vi "ESR Scanner - modified.vi"(0 "ESR Modified Parameters":T5={"Window 1 time (s)"=0.012, "Window 2 time (s)"=5e-06, "Window 3 time (s) "=0.02, "Window 4 time (s)"=5e-07, "Window 4 channels"=[TRUE, FALSE, FALSE, TRUE], "Window 3 channels"=[TRUE, FALSE, TRUE, TRUE], "Window 2 channels"=[TRUE, FALSE, FALSE, TRUE], "Window 1 channels"=[TRUE, TRUE, FALSE, TRUE], "Path to ESR Burner"=path "C:/Users/Loncar/Desktop/ESR VIs - Srujan/Sam Kim/PB/ESRFreq.exe", "Window 5 time (s)"=5e-07, "Drive channel"=0} {"Drive channel" max=8}, 1 "MW start freq (GHz)":dbl=2.84, 2 "MW stop freq (GHz)":dbl=2.9, 3 "# freq points":i32=61, 4 "# scans before track":i32=50, 5 "#scan iterations":i32=50, 6 "IntGraph Refnum":refnum<vi>, 7 "Optimize Parameters":T6={"Volt Step"={"X"=0.01, "Y"=0.01, "Z"=0.0}, "Num Iterations"=1, "Dwell Time (ms)"=100, "Volts Range"={"X"=0.1, "Y"=0.1, "Z"=0.0}, "Method"={"X"=enum."Max", "Y"=enum."Max", "Z"=enum."Max"}} {"Volts Range"."Z" min=0.0; "Volts Range"."Y" min=0.0; "Volts Range"."X" min=0.0; "Dwell Time (ms)" min=0; "Num Iterations" min=1 step=1; "Volt Step"."Z" min=1e-05; "Volt Step"."Y" min=1e-06; "Volt Step"."X" min=1e-06}, 8 "XY Graph Refnum":refnum<vi>, 9 "ESR Post-Processing Parameters":T3={"Cut-off Threshhold"=2.0, "Processing Type"=enum."Off"}, 10 "IntGraph Refnum 2":refnum<vi>, 11 "Data 1":T1={"Save avg spectrum graph?"=FALSE, "Path for avg spectrum graph"=path "C:/experiment/data/may_15_2012/SIL1_NV1_pippin_uW_off", "Save data to spreadsheet"=FALSE, "Path for avg spectrum spreadsheet"=path "C:/experiment/data/may_15_2012/SIL1_NV1_pippin_uW_off"}, 12 "XY Graph Refnum 2":refnum<vi>, 13 "Data 2":T2={"Save graph 2"=FALSE, "Path for avg spectrum graph 2"=path "C:/experiment/data/may_15_2012/SIL1_NV1_pippin_uW_off", "Save data to spreadsheet 2"=FALSE, "Path for avg spectrum spreadsheet 2"=path "C:/experiment/data/may_15_2012/SIL1_NV1_pippin_uW_off"}) -> ()   [LabVIEW 2012]
uses:
  Strict Type Def - Optimize Parameters Cluster.ctl
  ESR Modified Window Parameters.ctl
  ESR Processing Params.ctl
  ESR Processing State.ctl
  <vilib>/DAQmx/read.llb/DAQmx Read (Counter 1D U32 1Chan NSamp).vi
  Channels.vi
  <vilib>/DAQmx/miscellaneous.llb/DAQmx Fill In Error Info.vi
  Global Vars.vi
  <vilib>/Analysis/baseanly.llb/Mean (DBL).vi
  <vilib>/Utility/file.llb/Write To Spreadsheet File (DBL).vi
  <vilib>/Analysis/NI_AALBase.lvlib
panel:
  out "Counts vs. frequency 2":i32[][](graph)
  out "Avg ESR spectrum 2":cluster{"Y":dbl[], "Y":dbl[]}[](graph)
  out "Counts vs. frequency before processing":i32[][](graph)
  out "Counts vs. frequency":i32[][](graph)
  out "Avg ESR spectrum":cluster{"Y":dbl[], "Y":dbl[]}[](graph)
  # "Note:\nThis is not a standalone program. It is called from ScannerUI"
  # "Default PB connections:\nPB0 - MW switch\nPB1 - MW freq step\nPB2 - Counter sample clk\nPB3 - Green AOM"
  # "VI for ESR spectrum measurement\n08/26/2013, Srujan Meesala\n2/2/2015, Samuel Kim"
  # "Modified version:\nAlternates frequency sweep with channel on/off for driving cantilever"
  # "this is for each, ie 50 scans =\n50 scans off + 50 scans on"
  # "* <data>"
  # "MW freq step\ndwell time"
  # "MW freq step"
  # "Wait"
  # "Fluorescence\ncounting"
  # "Ctr sample clk"
  # "Wait"
  # "Wait between\nfreq sweeps"
  # "On/off between freq sweeps (off first)"
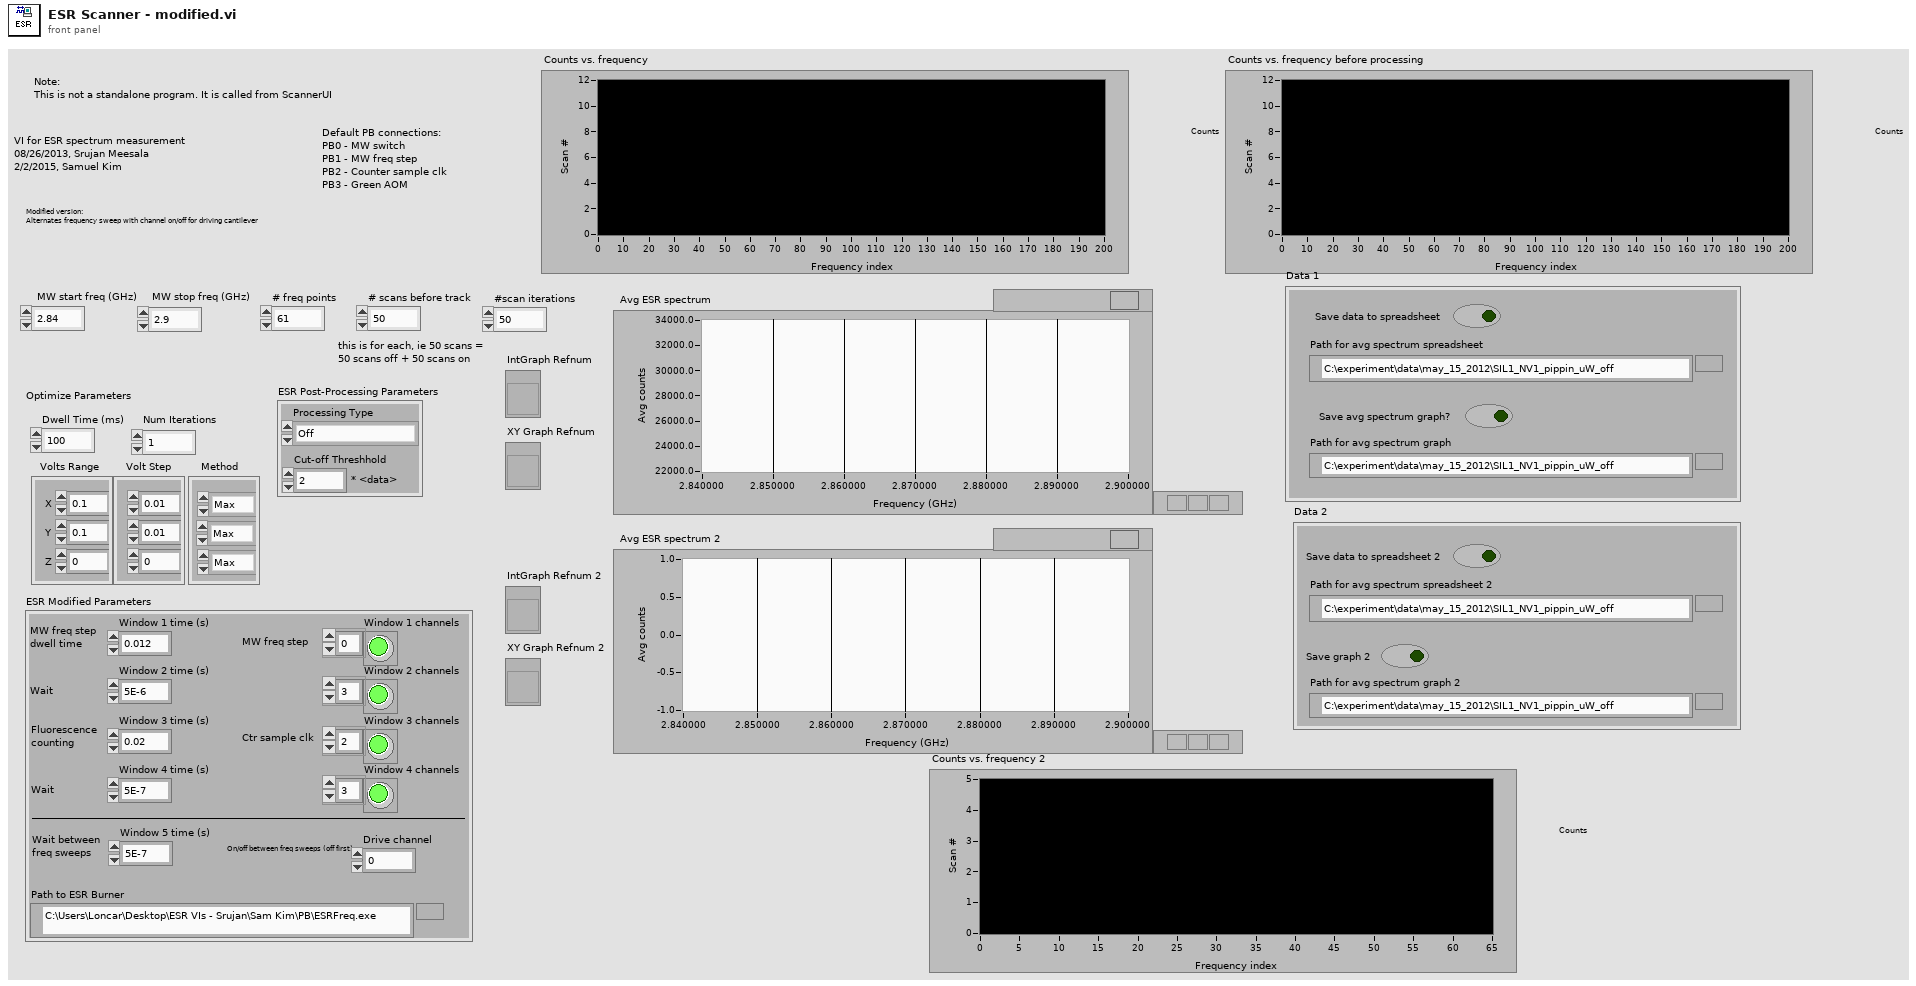
[diagram p1: front panel]
types:
  T1 = cluster{"Save avg spectrum graph?":bool, "Path for avg spectrum graph":path, "Save data to spreadsheet":bool, "Path for avg spectrum spreadsheet":path}
  T2 = cluster{"Save graph 2":bool, "Path for avg spectrum graph 2":path, "Save data to spreadsheet 2":bool, "Path for avg spectrum spreadsheet 2":path}
  T3 = typedef "ESR Processing Params.ctl" = cluster{"Cut-off Threshhold":dbl, "Processing Type":T4}
  T4 = typedef "ESR Processing State.ctl" = enum16{"Off", "Remove Outlier Scan", "Remove Outlier Data"}
  T5 = typedef "ESR Modified Window Parameters.ctl" = cluster{"Window 1 time (s)":dbl, "Window 2 time (s)":dbl, "Window 3 time (s) ":dbl, "Window 4 time (s)":dbl, "Window 4 channels":bool[], "Window 3 channels":bool[], "Window 2 channels":bool[], "Window 1 channels":bool[], "Path to ESR Burner":path, "Window 5 time (s)":dbl, "Drive channel":u8}
  T6 = typedef "Strict Type Def - Optimize Parameters Cluster.ctl" = cluster{"Volt Step":cluster{"X":dbl, "Y":dbl, "Z":dbl}, "Num Iterations":i32, "Dwell Time (ms)":i32, "Volts Range":cluster{"X":dbl, "Y":dbl, "Z":dbl}, "Method":cluster{"X":enum16{"Max", "Gaussian"}, "Y":enum16{"Max", "Gaussian"}, "Z":enum16{"Max", "Gaussian"}}}
  T7 = typedef "imagedata.ctl" = cluster{"image type":i32, "image depth":i32, "image":u8[], "mask":u8[], "colors":u32[], "Rectangle":cluster{"left":i16, "top":i16, "right":i16, "bottom":i16}}
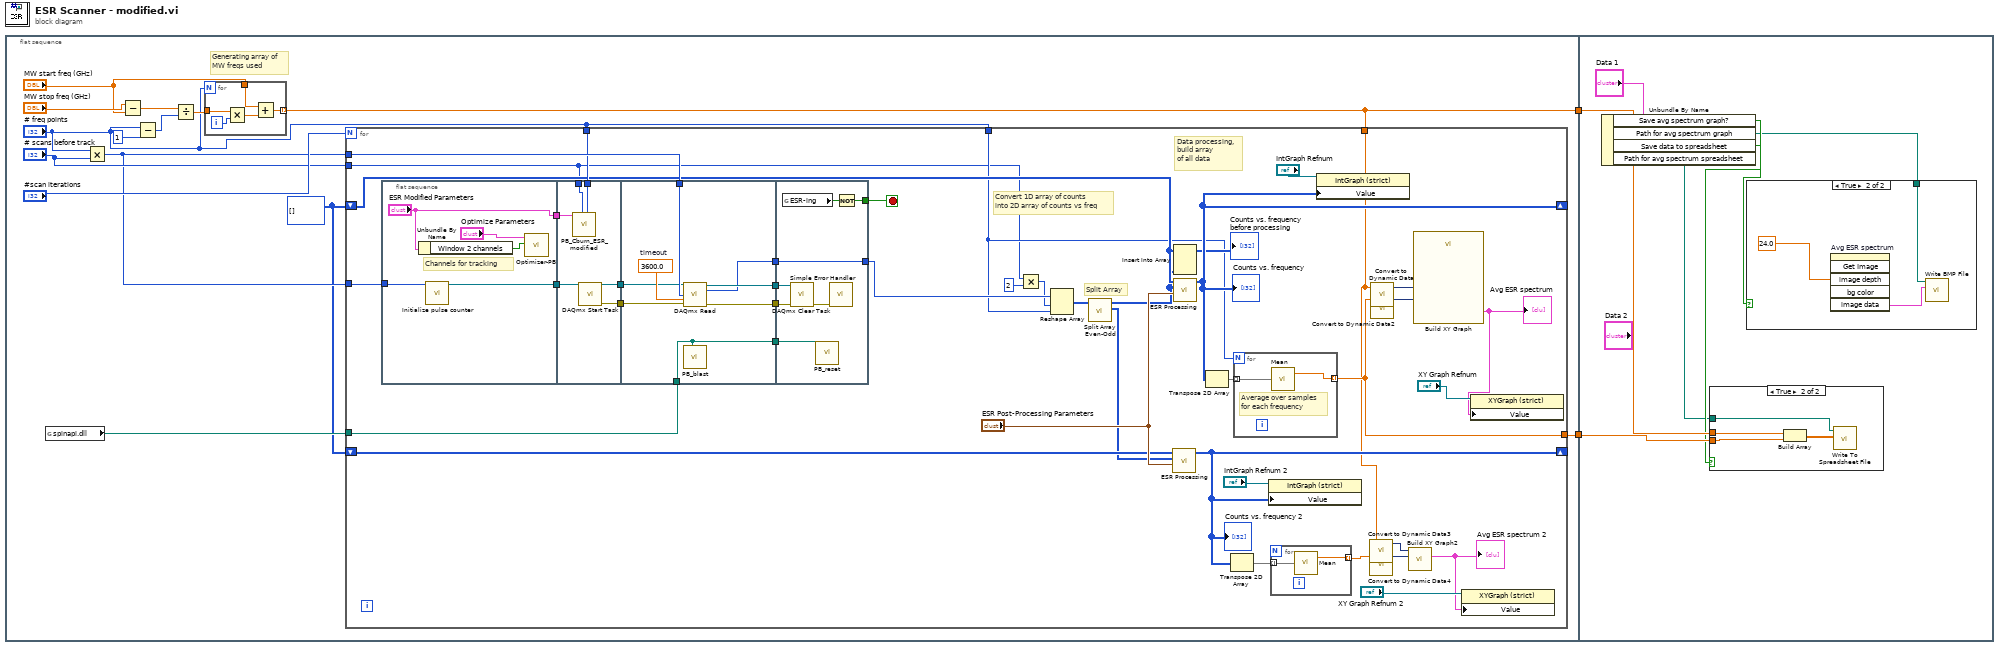
[diagram p0: block diagram]
diagram:
  n1 = flat-sequence {
    tunnel: [w9] -> w2
    tunnel: [w8] -> w1
    tunnel: w2 -> [w100]
    tunnel: w1 -> [w99]
    frame #0 {
      w3 = i32[][] [] ("Flourescence Data")
      # "Generating array of\nMW freqs used"
      n2 = global read "Channels.vi" "spinapi.dll"() -> (w6:path)
      n3 = Multiply(x="# freq points", y="# scans before track") -> (x*y=w4:i32)
      n4 = Subtract(x="MW stop freq (GHz)", y="MW start freq (GHz)") -> (x-y=w14:dbl)
      n5 = Subtract(x="# freq points", y=u32 1 ("Reset Count")) -> (x-y=w15:u32)
      n6 = Divide(x=w14, y=w15) -> (x/y=w12:dbl)
      n7 = for {
        N: "# freq points" -> [_]
        tunnel: w12 -> [w92]
        tunnel: "MW start freq (GHz)" -> [w90]
        tunnel: [w89] -> w9 mode=indexing
        i -> [w93]
        n8 = Multiply(x=w92, y=w93) -> (x*y=w91:dbl)
        n9 = Add(x=w90, y=w91) -> (x+y=w89:dbl)
      }
      n10 = for {
        N: "#scan iterations" -> [_]
        tunnel: w6 -> [w39]
        tunnel: w4 -> [w58]
        tunnel: "# scans before track" -> [w19]
        tunnel: "# freq points" -> [w23]
        shift-right: [w48] -> _
        shift-left: w3 -> [w37]
        tunnel: w9 -> [w29]
        tunnel: [w50] -> w8
        tunnel: "# freq points" -> [w44]
        tunnel: w4 -> [w41]
        shift-right: [w31] -> _
        shift-left: w3 -> [w34]
        stop <- w38 stop-if-true
        # "Split Array"
        # "Data processing,\nbuild array\nof all data"
        # "Convert 1D array of counts \ninto 2D array of counts vs freq"
        n11 = flat-sequence {
          tunnel: ["ESR Modified Parameters"] -> w45
          tunnel: w41 -> [w66]
          tunnel: [w65] -> w40
          tunnel: w45 -> [w68]
          tunnel: w19 -> [w70]
          tunnel: w44 -> [w69]
          tunnel: [w73] -> w43
          tunnel: [w72] -> w42
          tunnel: w40 -> [w71]
          tunnel: w58 -> [w80]
          tunnel: w39 -> [w77]
          tunnel: [w79] -> w57
          tunnel: [w78] -> w56
          tunnel: [w77] -> w55
          tunnel: [w74] -> w51
          tunnel: w43 -> [w76]
          tunnel: w42 -> [w75]
          tunnel: w57 -> [w85]
          tunnel: w56 -> [w86]
          tunnel: w55 -> [w88]
          tunnel: [w87] -> w24
          tunnel: w51 -> [w87]
          tunnel: [w82] -> w38
          frame #0 {
            # "Channels for tracking"
            n12 = Unbundle By Name("ESR Modified Parameters") -> ("Window 2 channels"=w64:bool[])
            n13 = call "Initialize pulse counter.vi"("Samples per channel"=w66) -> ("DAQmx Task Name"=w65:refnum<k21>)  [unwired: 9 in, 1 out]
            n14 = call "Optimizer-PB.vi"("Optimize active channels"=w64, "Optimize Parameters"="Optimize Parameters") -> ()  [unwired: 8 in, 2 out]
          }
          frame #1 {
            n15 = call "PB_Cburn_ESR_modified.vi"("# freq points"=w69, "# scans before track"=w70, "ESR Modified Parameters"=w68) -> ()  [unwired: 9 in]
            n16 = call <vilib>:"DAQmx Start Task.vi"("task/channels in"=w71) -> ("task out"=w73:refnum<k21>, "error out"=w72:errorcluster)  [unwired: 13 in]
          }
          frame #2 {
            w81 = 3600.0  # timeout
            n17 = call-poly <vilib>:"DAQmx Read.vi"("task/channels in"=w76, "number of samples per channel"=w80, "timeout"=w81, "error in"=w75) -> ("task out"=w78:refnum<k21>, "data"=w74:u32[], "error out"=w79:errorcluster)  [unwired: 9 in]
            n18 = call "PB_blast.vi"("Path to spinapi.dll"=w77) -> ()  [unwired: 7 in]
          }
          frame #3 {
            n19 = global read "Global Vars.vi" "ESR-ing"() -> (w83:bool)
            n20 = call <vilib>:"DAQmx Clear Task.vi"("task in"=w86, "error in"=w85) -> ("error out"=w84:errorcluster)  [unwired: 13 in]
            n21 = call "PB_reset.vi"("Path to spinapi.dll"=w88) -> ()  [unwired: 7 in]
            n22 = call <vilib>:"Simple Error Handler.vi"("error in (no error)"=w84) -> ()  [unwired: 4 in, 5 out]
            n23 = Not(x=w83) -> (.not. x?=w82:bool)
          }
        }
        n24 = Multiply(x=w19, y=2) -> (x*y=w17:i32)
        n25 = Reshape Array(w24, w17, w23) -> (w20:u32[][])
        n26 = call "Split Array Even-Odd.vi"("Input Array"=w20) -> ("Out Array 2"=w21:i32[][], "Out Array 1"=w22:i32[][])  [unwired: 9 in]
        n27 = call "ESR Processing.vi"("ESR Post-Processing Parameters"="ESR Post-Processing Parameters", "Array"=w21, "Flourescence Data in"=w34) -> ("Flourescence Data out"=w31:i32[][])  [unwired: 8 in]
        "Counts vs. frequency 2" <- w31
        n28 = Insert Into Array(array=w37, new element=w22) -> (→"Counts vs. frequency before processing":i32[][])  [unwired: 2 in]
        n29 = call "ESR Processing.vi"("ESR Post-Processing Parameters"="ESR Post-Processing Parameters", "Array"=w22, "Flourescence Data in"=w37) -> ("Flourescence Data out"=w48:i32[][])  [unwired: 8 in]
        "Counts vs. frequency" <- w48
        n30 = Transpose 2D Array(2D array=w48) -> (transposed array=w52:i32[][])
        n31 = Transpose 2D Array(2D array=w31) -> (transposed array=w32:i32[][])
        n32 = for {
          N: w23 -> [_]
          tunnel: [w62] -> w50 mode=indexing
          tunnel: w52 -> [w61] mode=indexing
          # "Average over samples\nfor each frequency"
          n33 = call-poly <vilib>:"Mean.vi"("X"=w61) -> ("mean"=w62:dbl)  [unwired: 1 out]
        }
        n34 = property class="IntGraph (strict)"(reference="IntGraph Refnum 2", "Value"=w31) -> ()  [unwired: 1 in, 2 out]
        n35 = for {
          tunnel: [w60] -> w27 mode=indexing
          tunnel: w32 -> [w59] mode=indexing
          n36 = call-poly <vilib>:"Mean.vi"("X"=w59) -> ("mean"=w60:dbl)  [unwired: 1 out]
        }
        n37 = property class="IntGraph (strict)"(reference="IntGraph Refnum", "Value"=w48) -> ()  [unwired: 1 in, 2 out]
        n38 = call "Convert to Dynamic Data3"("Array"=w29) -> ("Dynamic Data Type"=w28:dynamicdata)  [unwired: 3 in]
        n39 = call "Convert to Dynamic Data4"("Array"=w27) -> ("Dynamic Data Type"=w26:dynamicdata)  [unwired: 3 in]
        n40 = call "Convert to Dynamic Data"("Array"=w29) -> ("Dynamic Data Type"=w54:dynamicdata)  [unwired: 3 in]
        n41 = call "Convert to Dynamic Data2"("Array"=w50) -> ("Dynamic Data Type"=w53:dynamicdata)  [unwired: 3 in]
        n42 = call "Build XY Graph2"("Y Input"=w26, "X Input"=w28) -> ("XY Graph"=w25:cluster{"Y":dbl[], "Y":dbl[]}[])  [unwired: 3 in, 6 out]
        "Avg ESR spectrum 2" <- w25
        n43 = call "Build XY Graph"("Y Input"=w53, "X Input"=w54) -> ("XY Graph"=w46:cluster{"Y":dbl[], "Y":dbl[]}[])  [unwired: 3 in, 6 out]
        "Avg ESR spectrum" <- w46
        n44 = property class="XYGraph (strict)"(reference="XY Graph Refnum 2", "Value"=w25) -> ()  [unwired: 1 in, 2 out]
        n45 = property class="XYGraph (strict)"(reference="XY Graph Refnum", "Value"=w46) -> ()  [unwired: 1 in, 2 out]
      }
    }
    frame #1 {
      n46 = Unbundle By Name("Data 1") -> ("Save avg spectrum graph?"=w97:bool, "Path for avg spectrum graph"=w95:path, "Save data to spreadsheet"=w96:bool, "Path for avg spectrum spreadsheet"=w94:path)
      n47 = case shown="True" w96 {
        tunnel: w100 -> [_ w103]
        tunnel: w99 -> [_ w102]
        tunnel: w94 -> [_ w101]
        frame False {
        }
        frame True {
          n48 = Build Array(w103, w102) -> (w104:dbl[][])
          n49 = call-poly <vilib>:"Write To Spreadsheet File.vi"("2D data"=w104, "file path (dialog if empty)"=w101) -> ()  [unwired: 6 in, 1 out]
        }
      }
      n50 = case shown="True" w97 {
        tunnel: w95 -> [_ w105]
        frame False {
        }
        frame True {
          n51 = invoke on="Avg ESR spectrum" class="XYGraph (strict)" method="Get Image"("image depth"=24.0 ("Initial Delay")) -> ("image data"=w106:T7)  [unwired: 5 in, 5 out]
          n52 = call <vilib>:"Write BMP File.vi"("image data"=w106, "path to BMP file"=w105) -> ()  [unwired: 8 in, 2 out]
        }
      }
    }
  }
